vi "resetErrorCode.vi"(8 "error in (no error)":errorcluster, 11 "Model in":refnum<class "Model.lvclass">) -> (0 "error out":errorcluster, 3 "Model out":refnum<class "Model.lvclass">)   [LabVIEW 2012, in "Model.lvclass"]
uses:
  Model.lvclass
  Model.lvclass/Model.ctl
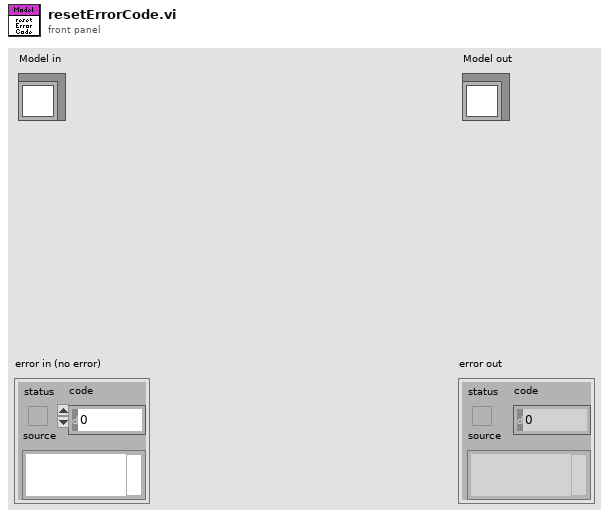
[diagram p1: front panel]
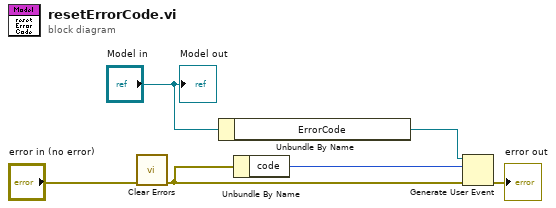
[diagram p0: block diagram]
diagram:
  n1 = call <vilib>:"Clear Errors.vi"("error in (no error)"="error in (no error)") -> ("error out"=w2:errorcluster)  [unwired: 6 in]
  n2 = Unbundle By Name("Model in") -> ("ErrorCode"=w5:refnum<user-event>)
  n3 = Unbundle By Name(w2) -> ("code"=w4:i32)
  n4 = Generate User Event(user event=w5, event data cluster=w4, error in=w2) -> (error out=→"error out":errorcluster)  [unwired: 1 out]
  "Model out" <- "Model in"
